vi "dequeue.vi"(8 "error in (no error)":errorcluster, 11 "manager_daemon in":refnum<class "manager_daemon.lvclass">) -> (0 "error out":errorcluster, 1 "data":variant, 2 "cmd":T1, 3 "manager_daemon out":refnum<class "manager_daemon.lvclass">)   [LabVIEW 2024, in "manager_daemon.lvclass"]
uses:
  manager_daemon.lvclass
  type_defs/cmd--enum.ctl
  manager_daemon.lvclass/manager_daemon.ctl
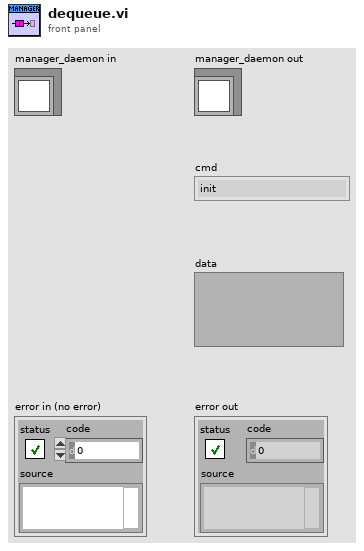
[diagram p1: front panel]
types:
  T1 = typedef "manager_daemon.lvclass/cmd--enum.ctl" = enum16{"init", "run", "load binaries", "build binaries", "save binaries", "display info", "apply filter", "add volume", "add issues", "add issue", "delete volume", "delete issues", "exit"}
  T2 = typedef "manager_daemon.lvclass/msg--cluster.ctl" = cluster{"cmd":T1, "data":variant}
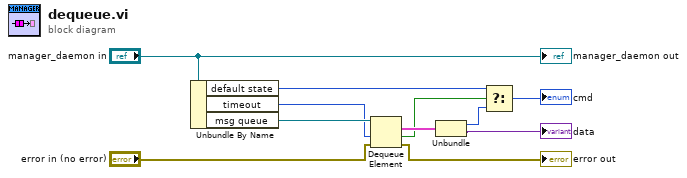
[diagram p0: block diagram]
diagram:
  n1 = Unbundle By Name("manager_daemon in") -> ("default state"=w4:T1, "timeout"=w9:i32, "msg queue"=w10:refnum<queue>)
  n2 = Dequeue Element(queue=w10, timeout in ms (-1)=w9, error in (no error)="error in (no error)") -> (element=w6:T2, timed out?=w5:bool, error out=→"error out":errorcluster)  [unwired: 1 out]
  n3 = Unbundle(w6) -> ("cmd"=w3:T1, "data"=→"data":variant)
  n4 = Select(t=w4, s=w5, f=w3) -> (s? t:f=→"cmd":T1)
  "manager_daemon out" <- "manager_daemon in"
